vi "Init.vi"(7 "CCWIsNegative":bool, 8 "error in (no error)":errorcluster, 9 "MaxRotation":dbl, 10 "PhysicalStepSize":dbl, 11 "StepperController in":refnum<class "StepperController.lvclass">) -> (0 "error out":errorcluster, 3 "StepperController out":refnum<class "StepperController.lvclass">)   [LabVIEW 2013, in "StepperController.lvclass"]
uses:
  StepperController.lvclass
  StepperController.lvclass/StepperController.ctl
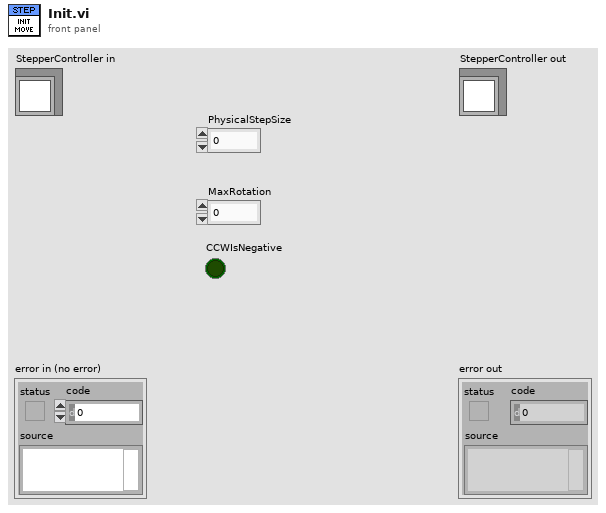
[diagram p1: front panel]
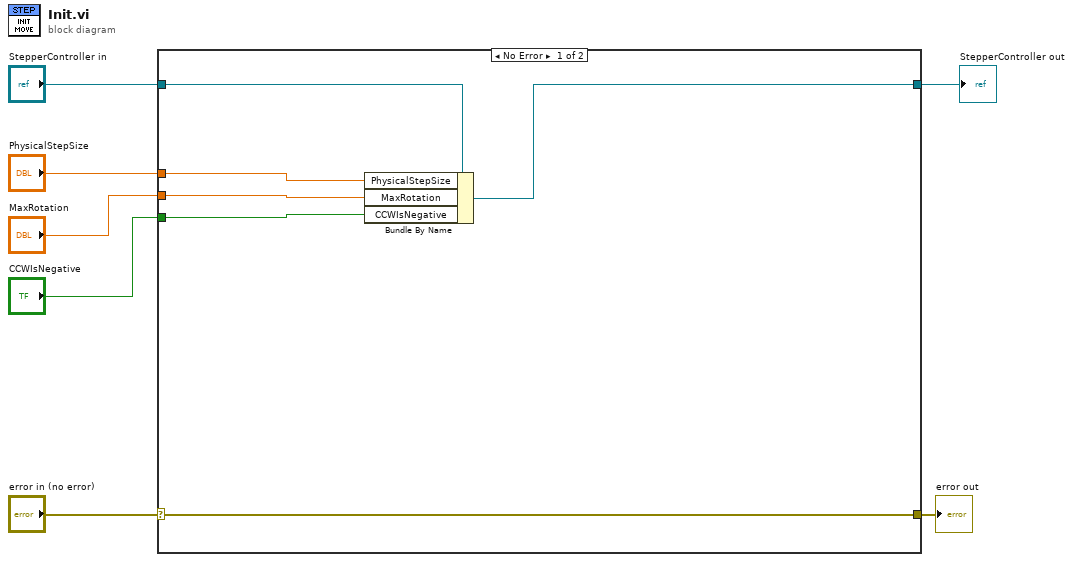
[diagram p0: block diagram]
diagram:
  n1 = case shown="No Error" "error in (no error)" {
    selector: "error in (no error)" -> [w13 w14]
    tunnel: [w13 w14] -> w6
    tunnel: [w11 w15] -> w1
    tunnel: "StepperController in" -> [w12 w15]
    tunnel: "PhysicalStepSize" -> [w10 _]
    tunnel: "MaxRotation" -> [w9 _]
    tunnel: "CCWIsNegative" -> [w8 _]
    frame No Error {
      n2 = Bundle By Name(cluster=w12, "PhysicalStepSize"=w10, "MaxRotation"=w9, "CCWIsNegative"=w8) -> (w11:refnum<class "StepperController.lvclass">)
    }
    frame Error {
    }
  }
  "error out" <- w6
  "StepperController out" <- w1
